vi "NI2564AOpenChannel.vi"(8 "error in (no error)":errorcluster, 10 "gRPCid":T4, 11 "HVC9 In":T1) -> (0 "error out":errorcluster, 3 "HVC9 Out":T1)   [LabVIEW 2019, in "HVC9 User.lvlib"]
uses:
  HVC9 User.lvlib
  Servers/HVC9/gRPC lvSupport/Server API/typeDefs/grpcId.ctl
  Types/HVC9.ctl
  Types/HVC9 gRPC IDs.ctl
  Types/HVC9 Data.ctl
  Servers/HVC9/HVC9 Class/RPC Messages/measurementservice_NI2564OpenChannelResponse/measurementservice_NI2564OpenChannelResponse_Data.ctl
  Servers/HVC9/HVC9 Class/RPC Messages/measurementservice_ErrorOut/measurementservice_ErrorOut_Data.ctl
  <instrlib>/niSwitch/niSwitch.llb/niSwitch Disconnect Channels (Single).vi
  Servers/HVC9/HVC9 Class/HVC9.lvclass
  Servers/HVC9/gRPC lvSupport/gprc-lvsupport.lvlib
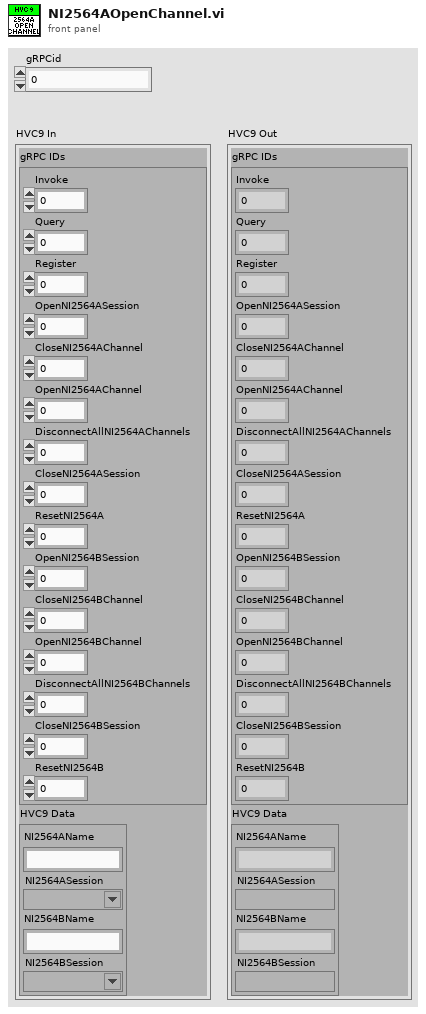
[diagram p1: front panel]
types:
  T1 = typedef "HVC9 User.lvlib/HVC9.ctl" = cluster{"gRPC IDs":T2, "HVC9 Data":T3}
  T2 = typedef "HVC9 User.lvlib/HVC9 gRPC IDs.ctl" = cluster{"Invoke ":u32, "Query":u32, "Register":u32, "OpenNI2564ASession":u32, "CloseNI2564AChannel ":u32, "OpenNI2564AChannel":u32, "DisconnectAllNI2564AChannels":u32, "CloseNI2564ASession":u32, "ResetNI2564A":u32, "OpenNI2564BSession":u32, "CloseNI2564BChannel ":u32, "OpenNI2564BChannel":u32, "DisconnectAllNI2564BChannels":u32, "CloseNI2564BSession":u32, "ResetNI2564B":u32}
  T3 = typedef "HVC9 User.lvlib/HVC9 Data.ctl" = cluster{"NI2564AName":string, "NI2564ASession":refnum<k15>, "NI2564BName":string, "NI2564BSession":refnum<k15>}
  T4 = typedef "HVC9.lvlib/gprc-lvsupport.lvlib/grpcId.ctl" = u64
  T5 = typedef "HVC9.lvlib/HVC9.lvclass/measurementservice_ErrorOut_Data.ctl" = cluster{"errCode":i32, "errMessage":string}
  T6 = typedef "HVC9.lvlib/HVC9.lvclass/measurementservice_NI2564OpenChannelResponse_Data.ctl" = cluster{"error":T5}
  T7 = typedef "HVC9.lvlib/HVC9.lvclass/measurementservice_NI2564OpenChannelRequest_Data.ctl" = cluster{"Channel1":string, "Channel2":string}
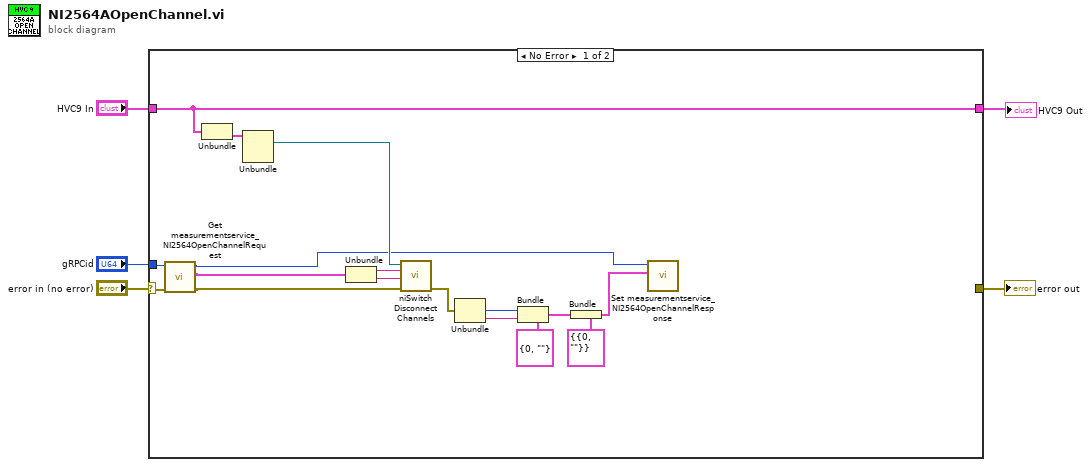
[diagram p0: block diagram]
diagram:
  n1 = case shown="No Error" "error in (no error)" {
    selector: "error in (no error)" -> [w9 w23]
    tunnel: [w20 w24] -> w1
    tunnel: "HVC9 In" -> [w20 w24]
    tunnel: "gRPCid" -> [w10 _]
    tunnel: [_ w23] -> w4
    frame No Error {
      n2 = call "Get measurementservice_NI2564OpenChannelRequest.vi"("error in (no error)"=w9, "gRPCid"=w10) -> ("error out"=w8:errorcluster, "Message Data"=w6:T7, "gRPCid out"=w7:T4)  [unwired: 7 in]
      n3 = Unbundle(w20) -> ("HVC9 Data"=w22:T3)  [unwired: 1 out]
      n4 = Unbundle(w22) -> ("NI2564ASession"=w21:refnum<k15>)  [unwired: 3 out]
      n5 = Unbundle(w6) -> ("Channel1"=w19:string, "Channel2"=w18:string)
      n6 = call-poly <instrlib>:"niSwitch Disconnect Channels.vi"("error in (no error)"=w8, "channel 2"=w18, "channel 1"=w19, "instrument handle"=w21) -> ("error out"=w14:errorcluster)  [unwired: 6 in, 1 out]
      n7 = Unbundle(w14) -> ("code"=w17:i32, "source"=w16:string)  [unwired: 1 out]
      n8 = Bundle(cluster=T5 {"errCode"=0, "errMessage"=""} ("error"), "errCode"=w17, "errMessage"=w16) -> (w11:T5)
      n9 = Bundle(cluster=T6 {"error"={"errCode"=0, "errMessage"=""}} ("measurementservice_NI2564OpenChannelResponse_Data"), "error"=w11) -> (w15:T6)
      n10 = call "Set measurementservice_NI2564OpenChannelResponse.vi"("Message Data"=w15, "gRPCid"=w7) -> ()  [unwired: 9 in, 1 out]
    }
    frame Error {
    }
  }
  "error out" <- w4
  "HVC9 Out" <- w1
